vi "circulo.vi.vi"() -> ()   [LabVIEW 2020]
panel:
  out "Circulo":cluster{dbl[], dbl[]}(graph)
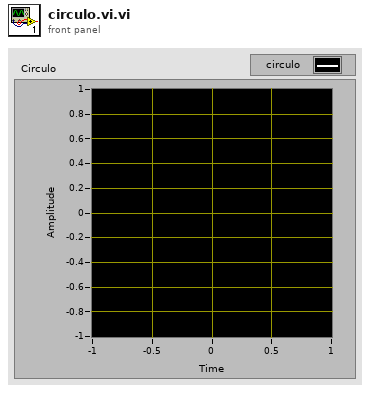
[diagram p1: front panel]
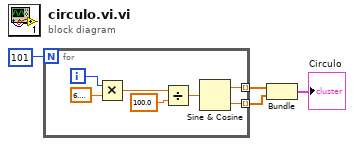
[diagram p0: block diagram]
diagram:
  n1 = for {
    N: 101 -> [_]
    tunnel: [w6] -> w4 mode=indexing
    tunnel: [w5] -> w3 mode=indexing
    i -> [w11]
    n2 = Multiply(x=w11, y=6.283185307179586) -> (x*y=w9:dbl)
    n3 = Divide(x=w9, y=100.0) -> (x/y=w8:dbl)
    n4 = Sine & Cosine(0:w8) -> (1:w6:dbl, 2:w5:dbl)
  }
  n5 = Bundle(w4, w3) -> (→"Circulo":cluster{dbl[], dbl[]})  [unwired: 1 in]
